vi "Set input trigger.vi"(8 "error in (no error)":errorcluster, 9 "Trigger mode":T1=1.0 items=["Normal"=1, "Start"=6], 10 "Trigger source":T2=1.0 items=["Internal"=1, "External"=2, "Software"=3], 11 "DAQOrcaFlash in":refnum<class "DAQOrcaFlash.lvclass">) -> (0 "error out":errorcluster, 3 "DAQOrcaFlash out":refnum<class "DAQOrcaFlash.lvclass">)   [LabVIEW 2012, in "DAQOrcaFlash.lvclass"]
uses:
  DAQOrcaFlash.lvclass
  trigger_source.ctl
  trigger_mode.ctl
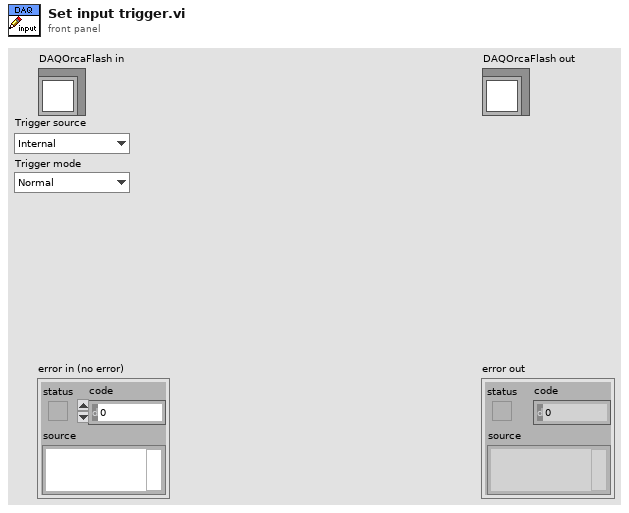
[diagram p1: front panel]
types:
  T1 = typedef "DAQOrcaFlash.lvclass/trigger_mode.ctl" = sgl
  T2 = typedef "DAQOrcaFlash.lvclass/trigger_source.ctl" = sgl
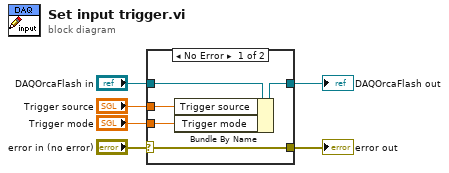
[diagram p0: block diagram]
diagram:
  n1 = case shown="No Error" "error in (no error)" {
    selector: "error in (no error)" -> [w11 w13]
    tunnel: [w11 w13] -> w5
    tunnel: [w9 w12] -> w3
    tunnel: "DAQOrcaFlash in" -> [w10 w12]
    tunnel: "Trigger source" -> [w8 _]
    tunnel: "Trigger mode" -> [w7 _]
    frame No Error {
      n2 = Bundle By Name(cluster=w10, "Trigger source"=w8, "Trigger mode"=w7) -> (w9:refnum<class "DAQOrcaFlash.lvclass">)
    }
    frame Error {
    }
  }
  "error out" <- w5
  "DAQOrcaFlash out" <- w3
